vi "Write address byte.vi"(8 "error in (no error)":errorcluster caption="에러 입력(에러 없음)", 10 "address byte":u8=1, 11 "I2C 입력":refnum<class "I2C.lvclass">) -> (0 "error out":errorcluster caption="에러 출력", 3 "I2C 출력":refnum<class "I2C.lvclass">)   [LabVIEW 2020, in "I2C.lvclass"]
uses:
  I2C.lvclass
  I2C.lvclass/I2C.ctl
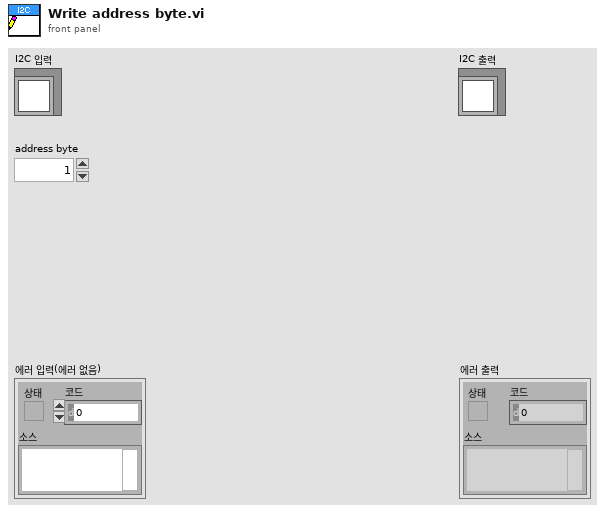
[diagram p1: front panel]
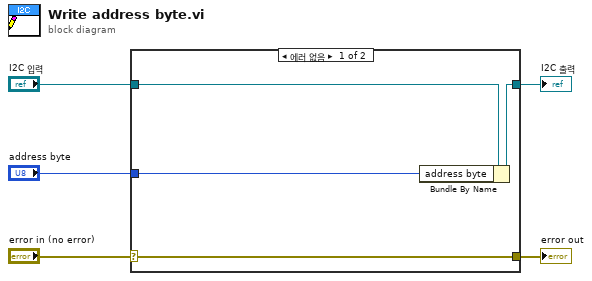
[diagram p0: block diagram]
diagram:
  n1 = case shown="에러 없음" "error in (no error)" {
    selector: "error in (no error)" -> [w9 w10]
    tunnel: [w9 w10] -> w4
    tunnel: [w7 w11] -> w2
    tunnel: "I2C 입력" -> [w8 w11]
    tunnel: "address byte" -> [w6 _]
    frame No Error {
      n2 = Bundle By Name(cluster=w8, "address byte"=w6) -> (w7:refnum<class "I2C.lvclass">)
    }
    frame Error {
    }
  }
  "error out" <- w4
  "I2C 출력" <- w2
